vi "Get Drive Information.vi"() -> (0 "Ticks/Revolution":dbl, 3 "Wheel Diameter":dbl)   [LabVIEW 2018]
doc: "Wheel diameter and encoder information for different drive bases. Useful for pathplanning."
panel:
  in  "Robot":enum16{"Vantage", "Mule"}(ring)
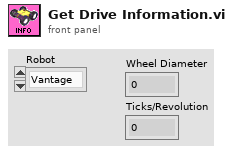
[diagram p1: front panel]
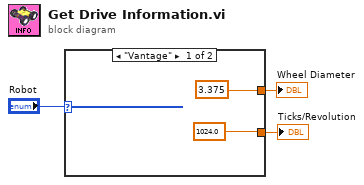
[diagram p0: block diagram]
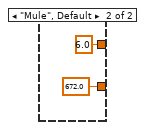
[diagram p2: hidden frame]
diagram:
  n1 = case shown="\"Vantage\"" "Robot" {
    tunnel: [3.375 ("x") 6.0 ("x")] -> w3
    tunnel: [1024.0 ("y") 672.0 ("y")] -> w2
    frame "Vantage" {
    }
    frame "Mule", Default {
    }
  }
  "Wheel Diameter" <- w3
  "Ticks/Revolution" <- w2
